vi "FOCUS_V42.vi"(9 "X-pixels":sgl=256.0, 11 "Run":bool) -> (0 "Retrace pixels":sgl, 10 "Pixel Clock (Hz)":sgl)   [LabVIEW 2010] (continued)
      n94 = local write "ScanLineFScope"(sgl[][] [[0.026666667, 0.10555588, 0.18413667, 0.2620946, 0.33912018, 0.4149288, 0.48917702, 0.5616217, 0.6319491, 0.69988036, 0.7651882, 0.8275282, 0.88674605, 0.9425593, 0.9947472, 1.043162, 1.087492, 1.127687, 1.163523, 1.1948596, 1.2216425, 1.2436236, 1.2608614, 1.2732126, 1.2806307, 1.2831601, 1.280641, 1.2732344, 1.2608918, 1.2436653, 1.2216938, 1.1949208, 1.1635948, 1.1277666, 1.0875816, 1.0432596, 0.9948533, 0.9426741, 0.8868671, 0.8276569, 0.7653226, 0.70002097, 0.6320957, 0.5617722, 0.48933217, 0.41508698, 0.33928153, 0.2622585, 0.18430196, 0.10572225, 0.026833316, -0.052056268, -0.13063815, -0.20859744, -0.28562555, -0.36143658, -0.43568876, -0.50813806, -0.57846946, -0.6464066, -0.71171933, -0.77406645, -0.833292, -0.8891114, -0.941308, -0.9897297, -1.0340693, -1.0742743, -1.110118, -1.1414653, -1.1682563, -1.1902486, -1.2074977, -1.2198576, -1.2272873, -1.2298253, -1.2273177, -1.2199228, -1.2075888, -1.1903737, -1.1684103, -1.1416483, -1.110333, -1.0745125, -1.0343375, -0.99002266, -0.9416256, -0.8894551, -0.83365417, -0.7744517, -0.71212274, -0.6468276, -0.57890815, -0.5085887, -0.43615317, -0.36191097, -0.28610873, -0.20908824, -0.13062674, -0.05199747], [-1.2831608, -1.2806358, -1.2732235, -1.2608767, -1.2436445, -1.2216686, -1.1948903, -1.163559, -1.1277268, -1.0875369, -1.0432112, -0.9948003, -0.94261676, -0.88680667, -0.8275926, -0.7652557, -0.69995075, -0.6320225, -0.56169707, -0.48925468, -0.41500804, -0.33920097, -0.26217666, -0.18421942, -0.105639175, -0.026750105, 0.052139297, 0.13072063, 0.20867924, 0.28570607, 0.3615159, 0.4357661, 0.5082131, 0.57854253, 0.6464767, 0.71178705, 0.7741306, 0.83335227, 0.88916856, 0.9413609, 0.9897791, 1.034114, 1.0743139, 1.1101538, 1.1414957, 1.1682826, 1.1902695, 1.2075129, 1.2198684, 1.2272923, 1.2298261, 1.2273127, 1.2199119, 1.2075737, 1.1903529, 1.1683854, 1.1416179, 1.1102973, 1.0744729, 1.034293, 0.98997456, 0.94157284, 0.889398, 0.833594, 0.7743877, 0.7120561, 0.6467577, 0.5788353, 0.50851387, 0.4360761, 0.3618324, 0.28602856, 0.20900682, 0.13105093, 0.052471776, -0.026417017, -0.10530679, -0.18388921, -0.2618492, -0.33887854, -0.4146908, -0.48894495, -0.56139654, -0.63172984, -0.69966996, -0.76498514, -0.82733583, -0.8865652, -0.94238764, -0.9945887, -1.0430137, -1.0873581, -1.127568, -1.1634157, -1.1947683, -1.2215633, -1.2435613, -1.260816, -1.2693994, -1.2762786]] ("transposed array")) -> ()
    }
  }
  n95 = Type Cast(type="" ("name or relative path"), x=w48) -> (*(type *) &x=w45:string)
  n96 = Type Cast(type=tag "" ("6229 Device 2"), x=w65) -> (*(type *) &x=w64:tag)
  n97 = Type Cast(type=refnum<visa-resource-name> " " ("VISA Sutter MP-285"), x=w50) -> (*(type *) &x=w49:refnum<visa-resource-name>)
  n98 = Type Cast(type=refnum<visa-resource-name> refnum ("VISA Sutter MP-285"), x=w54) -> (*(type *) &x=w4:refnum<visa-resource-name>)
  n99 = property on="Run" class="Bool (strict)"("Visible"=w100) -> ()  [unwired: 2 in, 2 out]
  n100 = local write "End experiment"(w101) -> ()
  n101 = property on="colour table" class="Arr (strict)"("Value"=w37) -> ()  [unwired: 2 in, 2 out]
  n102 = property on="Galvos" class="XYGraph (strict)"("X Scale.Range:Minimum"=w3, "X Scale.Range:Maximum"="Scangraph scaling", "Y Scale.Range:Minimum"=w2, "Y Scale.Range:Maximum"="Scangraph scaling") -> ()  [unwired: 2 in, 2 out]
  n103 = Type Cast(type=u16 0 ("Program Version"), x=w84) -> (*(type *) &x=→"Program Version":u16)
  n104 = String To Path(string=w45) -> (path=w44:path)
  n105 = local write "FocusModeSelector"(TRUE ("FocusModeSelector")) -> ()
  n106 = local write "new FreeLine?"(FALSE ("new udl?")) -> ()
  n107 = local write "NewScanpattern"(FALSE ("NewScanpattern")) -> ()
  n108 = local write "VISA XPG-ADC"(w49) -> ()
  n109 = local write "AO/DIO Device"(w67) -> ()
  n110 = local write "VISA Sutter MP-285"(w4) -> ()
  n111 = property on="stop 2" class="Bool (strict)"("Visible"=w100) -> ()  [unwired: 2 in, 2 out]
  n112 = property on="Scan format" class="Ring (strict)"("Disabled"=u8 0) -> ()  [unwired: 2 in, 2 out]
  n113 = local write "AI Device"(w64) -> ()
  n114 = local write "MaiTai setting Path"(w44) -> ()
  n115 = local write "reset?"(125.0 ("reset?")) -> ()
  n116 = property on="Image 2" class="IntGraph (strict)"("Color Table"=w37) -> ()  [unwired: 2 in, 2 out]
  n117 = property on="End experiment" class="Bool (strict)"("Visible"=w100) -> ()  [unwired: 2 in, 2 out]
  n118 = local write "stop 2"(w101) -> ()
  n119 = property on="Hit Graph" class="IntGraph (strict)"("Color Table"=w37) -> ()  [unwired: 2 in, 2 out]
  n120 = while {
    tunnel: w6 -> [w206]
    tunnel: [w161] -> w5
    stop <- w162 stop-if-true
    n121 = flat-sequence {
      tunnel: [w1452] -> w294
      tunnel: w294 -> [w1667]
      tunnel: [w1625] -> w176
      tunnel: [w1640] -> w174
      tunnel: ["Zoom 1 scan voltage"] -> w173
      tunnel: [w1637] -> w172
      tunnel: [w1636] -> w171
      tunnel: [w1621] -> w169
      tunnel: [w1620] -> w168
      tunnel: [w2016] -> w258
      tunnel: [w2015] -> w287
      tunnel: [w1901] -> w289
      tunnel: [w2007] -> w259
      tunnel: [w1962] -> w297
      tunnel: [w1955] -> w261
      tunnel: [w1922] -> w296
      tunnel: [w2013] -> w260
      tunnel: [w2012] -> w284
      tunnel: [w2037] -> w282
      tunnel: [w2030] -> w281
      tunnel: w175 -> [w1886]
      tunnel: w185 -> [w1885]
      tunnel: [w1884] -> w181
      tunnel: w176 -> [w1872]
      tunnel: w174 -> [w1858]
      tunnel: w173 -> [w1871]
      tunnel: w172 -> [w1870]
      tunnel: w171 -> [w1869]
      tunnel: w170 -> [w1867]
      tunnel: w169 -> [w1863]
      tunnel: w168 -> [w1862]
      tunnel: [w1859] -> w167
      frame #0 {
        n122 = property on="Fiberscope" class="TabCtl (strict)"("Visible"="Fiberscope\nMode") -> ()  [unwired: 2 in, 2 out]
        n123 = property on="Hit Graph" class="IntGraph (strict)"("Visible"="Fiberscope\nMode") -> ()  [unwired: 2 in, 2 out]
        n124 = property on="Scale" class="Slide (strict)"("Visible"="Fiberscope\nMode") -> ()  [unwired: 2 in, 2 out]
        n125 = case shown="False" "Fiberscope\nMode" {
          tunnel: ["Mode selector" "Mode selectorFScope"] -> w1452
          frame False {
            n126 = case shown="0, Default" "Scan format" {
              tunnel: [w1558 sgl 64.0 ("X-pixels") sgl 128.0 ("X-pixels") sgl 256.0 ("X-pixels") sgl 512.0 ("X-pixels") sgl 32.0 ("X-pixels")] -> w1483
              tunnel: [w1557 sgl 64.0 ("Y-lines") sgl 128.0 ("Y-lines") sgl 256.0 ("Y-lines") sgl 512.0 ("Y-lines") sgl 32.0 ("Y-lines")] -> w1482
              tunnel: [w1556 sgl 2.0 ("line scan time (ms)") sgl 2.0 ("line scan time (ms)") sgl 2.0 ("line scan time (ms)") sgl 2.0 ("line scan time (ms)") sgl 1.0 ("line scan time (ms)")] -> w1481
              tunnel: [0 2 2 2 2 2] -> w1480
              frame 0, Default {
                n127 = local read "line scan time (ms)"() -> (w1556:sgl)
                n128 = local read "X-pixels"() -> (w1558:sgl)
                n129 = local read "Y-lines"() -> (w1557:sgl)
              }
              frame 1 {
              }
              frame 2 {
              }
              frame 3 {
              }
              frame 4 {
              }
              frame 5 {
              }
            }
            n130 = case shown="0, Default" "Mode selector" {
              tunnel: [2 0 2 2 0 2] -> w1464
              tunnel: [0 1 2 3 1 4] -> w1474
              tunnel: [w1495 w1505 0 w1526 w1536 w1546] -> w1470
              tunnel: w1480 -> [w1495 w1505 _ _ w1536 _]
              tunnel: [0 0 2 2 0 2] -> w1465
              tunnel: [w1500 w1510 u16 0 ("Scan format") u16 0 ("Scan format") w1541 u16 0 ("Scan format")] -> w1479
              tunnel: [TRUE ("Visible") FALSE ("Visible") FALSE ("Visible") FALSE ("Visible") FALSE ("Visible") FALSE ("Visible")] -> w1472
              tunnel: [u8 2 ("Disabled") u8 2 ("Disabled") u8 2 ("Disabled") u8 0 ("Disabled") u8 2 ("Disabled") u8 0 ("Disabled")] -> w1469
              tunnel: [2 2 2 2 2 0] -> w1460
              tunnel: [2 0 0 2 0 2] -> w1463
              tunnel: [w1495 w1505 2 w1526 w1536 w1546] -> w1462
              tunnel: [u8 2 ("Disabled") u8 2 ("Disabled") u8 0 ("Disabled") u8 0 ("Disabled") u8 2 ("Disabled") u8 2 ("Disabled")] -> w1461
              frame 0, Default {
                # "Focus mode"
                n131 = local read "Scan format"() -> (w1500:u16)
              }
              frame 1 {
                # "frame scan"
                n132 = local read "Scan format"() -> (w1510:u16)
              }
              frame 2 {
                # "straight line scan"
              }
              frame 3 {
                w1526 = 2
                # "user-defined line"
              }
              frame 4 {
                # "frame scan piezo"
                n133 = local read "Scan format"() -> (w1541:u16)
              }
              frame 5 {
                w1546 = 2
                # "user-defined line 3D"
              }
            }
            "frame/line indicator" <- w1474
            n134 = Less?(x=w1474, y=u16 3) -> (x < y?=w1476:bool)
            n135 = case shown="False" w1476 {
              tunnel: [TRUE ("Visible") FALSE ("Visible")] -> w1475
              tunnel: [w1487 FALSE ("Visible")] -> w1471
              frame False {
                n136 = property on="Image 3" class="IntGraph (strict)"() -> ("Visible"=w1487:bool)  [unwired: 2 in, 2 out]
              }
              frame True {
              }
            }
            n137 = case shown="3" "Scan format 2" {
              tunnel: [i16 10 ("X-pixels") i16 20 ("X-pixels") i16 40 ("X-pixels") i16 60 ("X-pixels")] -> w1467
              frame 0, Default {
              }
              frame 1 {
              }
              frame 2 {
              }
              frame 3 {
              }
            }
            n138 = local write "X-pixels"(w1483) -> ()
            n139 = local write "Y-lines"(w1482) -> ()
            n140 = local write "line scan time (ms)"(w1481) -> ()
            n141 = property on="phase shift [°]" class="DigNum (strict)"("Disabled"=w1460) -> ()  [unwired: 2 in, 2 out]
            n142 = local write "Scan format"(w1479) -> ()
            n143 = property on="Number of frames" class="DigNum (strict)"("Disabled"=w1463) -> ()  [unwired: 2 in, 2 out]
            n144 = property on="Averaging" class="DigNum (strict)"("Disabled"=w1464) -> ()  [unwired: 2 in, 2 out]
            n145 = property on="z-step (um)" class="DigNum (strict)"("Disabled"=w1464) -> ()  [unwired: 2 in, 2 out]
            n146 = property on="Scan format" class="Ring (strict)"("Disabled"=w1465) -> ()  [unwired: 2 in, 2 out]
            n147 = property on="X-pixels" class="DigNum (strict)"("Disabled"=w1470) -> ()  [unwired: 2 in, 2 out]
            n148 = property on="#" class="DigNum (strict)"("Disabled"=w1470) -> ()  [unwired: 2 in, 2 out]
            n149 = property on="line scan time (ms)" class="DigNum (strict)"("Disabled"=w1470) -> ()  [unwired: 2 in, 2 out]
            n150 = property on="#" class="DigNum (strict)"("Disabled"=w1469) -> ()  [unwired: 2 in, 2 out]
            n151 = property on="Y-lines FreeLine" class="DigNum (strict)"("Disabled"=w1469) -> ()  [unwired: 2 in, 2 out]
            n152 = property on="Y-Scale" class="Bool (strict)"("Disabled"=w1461) -> ()  [unwired: 2 in, 2 out]
            n153 = local write "ImageSelector"(w1471) -> ()
            n154 = property on="XY Graph 1" class="XYGraph (strict)"("Visible"=w1475) -> ()  [unwired: 2 in, 2 out]
            n155 = property on="XY Graph 2" class="XYGraph (strict)"("Visible"=w1475) -> ()  [unwired: 2 in, 2 out]
            n156 = property on="Image 3" class="IntGraph (strict)"("Visible"=w1471) -> ()  [unwired: 2 in, 2 out]
            n157 = property on="Histogram1" class="XYGraph (strict)"("Visible"=w1471) -> ()  [unwired: 2 in, 2 out]
            n158 = property on="Y-lines" class="DigNum (strict)"("Disabled"=w1462) -> ()  [unwired: 2 in, 2 out]
            n159 = Divide(x=4000.0, y=w1467) -> (x/y=→"pixelstoµm":dbl)
            n160 = property on="FocusModeSelector" class="Bool (strict)"("Visible"=w1472) -> ()  [unwired: 2 in, 2 out]
            n161 = property on="XY Graph 3" class="XYGraph (strict)"("Visible"=FALSE) -> ()  [unwired: 2 in, 2 out]
            n162 = property on="XY Graph 4" class="XYGraph (strict)"("Visible"=w1475) -> ()  [unwired: 2 in, 2 out]
            n163 = property on="Image 4" class="IntGraph (strict)"("Visible"=w1471) -> ()  [unwired: 2 in, 2 out]
            n164 = property on="Amplitude Factor" class="DigNum (strict)"("Disabled"=w1460) -> ()  [unwired: 2 in, 2 out]
            n165 = property on="z frequency" class="Slide (strict)"("Disabled"=w1460) -> ()  [unwired: 2 in, 2 out]
            n166 = property on="Histogram2" class="XYGraph (strict)"("Visible"=w1471) -> ()  [unwired: 2 in, 2 out]
            n167 = local write "Open?"(FALSE ("Open?")) -> ()
            n168 = property on="new FreeLine?" class="Bool (strict)"("Disabled"=w1469) -> ()  [unwired: 2 in, 2 out]
            n169 = property on="#" class="DigNum (strict)"("Disabled"=w1463) -> ()  [unwired: 2 in, 2 out]
            n170 = property on="#" class="DigNum (strict)"("Disabled"=w1464) -> ()  [unwired: 2 in, 2 out]
            n171 = property on="Time interval [s]" class="DigNum (strict)"("Disabled"=w1464) -> ()  [unwired: 2 in, 2 out]
            n172 = property on="Number of stacks" class="DigNum (strict)"("Disabled"=w1464) -> ()  [unwired: 2 in, 2 out]
            n173 = property on="#" class="DigNum (strict)"("Disabled"=w1464) -> ()  [unwired: 2 in, 2 out]
            n174 = property on="Cusp Delay" class="DigNum (strict)"("Disabled"=w1465) -> ()  [unwired: 2 in, 2 out]
          }
          frame True {
            n175 = local write "Mode selector"("Mode selectorFScope") -> ()
            n176 = case shown="0, Default" "Mode selectorFScope" {
              tunnel: [u16 2 ("Mode selectorFScope") u16 0 ("Mode selectorFScope") u16 2 ("Mode selectorFScope")] -> w1579
              tunnel: [u16 0 ("Mode selectorFScope") u16 0 ("Mode selectorFScope") u16 2 ("Mode selectorFScope")] -> w1582
              tunnel: [w1593 w1596 u16 0 ("Scan format FScope")] -> w1581
              frame 0, Default {
                n177 = local read "Scan format FScope"() -> (w1593:u16)
              }
              frame 1 {
                n178 = local read "Scan format FScope"() -> (w1596:u16)
              }
              frame 2 {
              }
            }
            n179 = local write "frame/line indicator"("Mode selectorFScope") -> ()
            n180 = local write "Time interval [s]"("Time interval [s]") -> ()
            n181 = local write "Number of stacks"("Number of Stacks") -> ()
            n182 = local read "Number of Frames"() -> (w1588:sgl)
            n183 = case shown="0, Default" "Scan format FScope" {
              tunnel: [w1604 sgl 64.0 ("X dim") sgl 128.0 ("X dim") sgl 256.0 ("X dim") sgl 512.0 ("X dim") sgl 32.0 ("X dim")] -> w1590
              tunnel: [w1603 sgl 64.0 ("Y dim") sgl 128.0 ("Y dim") sgl 256.0 ("Y dim") sgl 512.0 ("Y dim") sgl 32.0 ("Y dim")] -> w1589
              tunnel: [u8 0 ("Disabled") u8 2 ("Disabled") u8 2 ("Disabled") u8 2 ("Disabled") u8 2 ("Disabled") u8 2 ("Disabled")] -> w1591
              frame 0, Default {
                n184 = local read "Y dim"() -> (w1603:sgl)
                n185 = local read "X dim"() -> (w1604:sgl)
              }
              frame 1 {
              }
              frame 2 {
              }
              frame 3 {
              }
              frame 4 {
              }
              frame 5 {
              }
            }
            n186 = local read "Averaging"() -> (w1587:sgl)
            n187 = local write "Scan format FScope"(w1581) -> ()
            n188 = property on="Scan format FScope" class="Ring (strict)"("Disabled"=w1582) -> ()  [unwired: 2 in, 2 out]
            n189 = property on="Time interval [s]" class="DigNum (strict)"("Disabled"=w1579) -> ()  [unwired: 2 in, 2 out]
            n190 = property on="Number of Stacks" class="DigNum (strict)"("Disabled"=w1579) -> ()  [unwired: 2 in, 2 out]
            n191 = property on="Number of Frames" class="DigNum (strict)"("Disabled"=w1579) -> ()  [unwired: 2 in, 2 out]
            n192 = property on="Averaging" class="DigNum (strict)"("Disabled"=w1579) -> ()  [unwired: 2 in, 2 out]
            n193 = property on="#" class="DigNum (strict)"("Disabled"=w1579) -> ()  [unwired: 2 in, 2 out]
            n194 = property on="#" class="DigNum (strict)"("Disabled"=w1579) -> ()  [unwired: 2 in, 2 out]
            n195 = property on="#" class="DigNum (strict)"("Disabled"=w1579) -> ()  [unwired: 2 in, 2 out]
            n196 = local write "X dim"(w1590) -> ()
            n197 = local write "Y dim"(w1589) -> ()
            n198 = property on="Y dim" class="DigNum (strict)"("Disabled"=w1591) -> ()  [unwired: 2 in, 2 out]
            n199 = local write "Number of frames"(w1588) -> ()
            n200 = local write "Averaging"(w1587) -> ()
            n201 = global write "GlobelFSCOPE.vi" "X dim"(w1590) -> ()
            n202 = global write "GlobelFSCOPE.vi" "Y dim"(w1589) -> ()
            n203 = property on="X dim" class="DigNum (strict)"("Disabled"=w1591) -> ()  [unwired: 2 in, 2 out]
            n204 = local write "X-pixels"("X dim") -> ()
            n205 = local write "Y-lines"("Y dim") -> ()
            n206 = global write "GlobelFSCOPE.vi" "Y dim"("Y dim") -> ()
            n207 = global write "GlobelFSCOPE.vi" "X dim"("X dim") -> ()
          }
        }
        n208 = local read "GetFirst"() -> (w1446:bool)
        n209 = local read "GetLast"() -> (w1445:bool)
        n210 = And(x=w1446, y=w1445) -> (x .and. y?=w1444:bool)
        n211 = case shown="True" w1444 {
          frame False {
          }
          frame True {
            n212 = local read "Number of frames"() -> (w1456:sgl)
            n213 = local read "FirstPosition"() -> (w1453:sgl)
            n214 = local read "LastPosition"() -> (w1454:sgl)
            n215 = Decrement(x=w1456) -> (x-1=w1457:sgl)
            n216 = Subtract(x=w1454, y=w1453) -> (x-y=w1458:sgl)
            n217 = Divide(x=w1458, y=w1457) -> (x/y=w1455:sgl)
            n218 = local write "z-step (um)"(w1455) -> ()
          }
        }
        n219 = Get Date/Time String(date format (0)=enum16{"short", "long", "abbreviated"}."abbreviated") -> (time string=→"Time":string)  [unwired: 2 in, 1 out]
        n220 = Format Date/Time String(time format string (%c)="%m%d%y") -> (date/time string=→"Date":string)  [unwired: 2 in]
      }
      frame #1 {
        # "Line scan position and measurement cursors"
        n221 = local read "frame/line indicator"() -> (w1640:u16)
        n222 = Less?(x=w1667, y=3.0) -> (x < y?=w1662:bool)
        n223 = And(x="View line\ncheck box", y=w1662) -> (x .and. y?=w1666:bool)
        n224 = And(x=w1662, y="Measurement cursor check box") -> (x .and. y?=w1661:bool)
        n225 = control-ref of="Image 2"() -> (w1664:refnum<vi>)
        n226 = control-ref of="Image 1"() -> (w1665:refnum<vi>)
        n227 = Divide(x="Y-lines", y="X-pixels") -> (x/y=w1670:sgl)
        n228 = case "Measurement cursor on/off" shown="True" w1661 {
          tunnel: w1664 -> [w1744 w1750]
          tunnel: w1665 -> [w1745 w1751]
          frame False {
            w1743 = FALSE ("Cursor.Visible")
            w1746 = u32 1 ("Active Cursor")
            n229 = property on="OGB value" class="DigNum (strict)"("Visible"=w1743) -> ()  [unwired: 2 in, 2 out]
            n230 = property on="Alexa value" class="DigNum (strict)"("Visible"=w1743) -> ()  [unwired: 2 in, 2 out]
            n231 = property on="Property Node" class="IntGraph (strict)"(reference=w1745, "Active Cursor"=w1746, "Cursor.Visible"=w1743) -> ()  [unwired: 1 in, 2 out]
            n232 = property on="Property Node" class="IntGraph (strict)"(reference=w1744, "Active Cursor"=w1746, "Cursor.Visible"=w1743) -> ()  [unwired: 1 in, 2 out]
          }
          frame True {
            w1747 = u32 1 ("Active Cursor")
            w1752 = u32 16776960
            w1748 = TRUE ("Cursor.Visible")
            w1753 = u32 1 ("Active Cursor")
            n233 = while {
              tunnel: w1751 -> [w1764]
              tunnel: w1750 -> [w1763]
              stop <- w1754 continue-if-true
              w1762 = u32 1 ("Active Cursor")
              n234 = property on="Property Node" class="IntGraph (strict)"(reference=w1764, "Active Cursor"=w1762) -> ("Cursor.Cursor Position:Cursor X"=w1758:dbl, "Cursor.Cursor Position:Cursor Y"=w1756:dbl, "Value"=w1761:u8[][])  [unwired: 1 in, 2 out]
              n235 = Index Array(array=w1761, index (row)=w1758, index (col)=w1756) -> (element=→"OGB value":u8)
              n236 = property on="Property Node" class="IntGraph (strict)"(reference=w1763, "Active Cursor"=w1762, "Cursor.Cursor Position:Cursor X"=w1758, "Cursor.Cursor Position:Cursor Y"=w1756) -> ("Value"=w1757:u8[][])  [unwired: 1 in, 2 out]
              n237 = Index Array(array=w1757, index (row)=w1758, index (col)=w1756) -> (element=→"Alexa value":u8)
              n238 = local read "Measurement cursor check box"() -> (w1755:bool)
              n239 = case shown="False" w1755 {
                selector: w1755 -> [w1765 w1767]
                tunnel: [w1765 w1767] -> w1754
                frame False {
                  n240 = property on="Run" class="Bool (strict)"("Disabled"=u8 0) -> ()  [unwired: 2 in, 2 out]
                }
                frame True {
                }
              }
            }
            n241 = property on="Run" class="Bool (strict)"("Disabled"=u8 2) -> ()  [unwired: 2 in, 2 out]
            n242 = property on="Property Node" class="IntGraph (strict)"(reference=w1751, "Active Cursor"=w1753, "Cursor.Visible"=w1748, "Cursor.Cursor Color"=w1752, "Cursor.Cursor Position:Cursor X"=w1747, "Cursor.Cursor Position:Cursor Y"=w1747) -> ()  [unwired: 1 in, 2 out]
            n243 = property on="Property Node" class="IntGraph (strict)"(reference=w1750, "Active Cursor"=w1753, "Cursor.Visible"=w1748, "Cursor.Cursor Color"=w1752) -> ()  [unwired: 1 in, 2 out]
            n244 = property on="OGB value" class="DigNum (strict)"("Visible"=w1748) -> ()  [unwired: 2 in, 2 out]
            n245 = property on="Alexa value" class="DigNum (strict)"("Visible"=w1748) -> ()  [unwired: 2 in, 2 out]
          }
        }
        n246 = Greater?(x=w1670, y=1.0) -> (0:w1671:bool)
        n247 = local read "Fiberscope\nMode"() -> (w1645:bool)
        n248 = case shown="True" w1645 {
          tunnel: [w1684 w1685] -> w1659
          frame False {
            n249 = local read "Mode selector"() -> (w1684:u16)
          }
          frame True {
            n250 = local read "Mode selectorFScope"() -> (w1685:u16)
          }
        }
        n251 = case shown="False" w1671 {
          tunnel: w1670 -> [w1774 _]
          tunnel: [w1773 w1813] -> w1653
          tunnel: [w1771 w1812] -> w1652
          tunnel: [w1770 w1811] -> w1651
          frame False {
            w1769 = u32 512 ("Plot Area:Size:Width")
            n252 = Multiply(x=w1769, y=w1774) -> (x*y=w1768:sgl)
            n253 = property on="Image 1" class="IntGraph (strict)"("Plot Area:Size:Width"=w1769, "Plot Area:Size:Height"=w1768) -> ()  [unwired: 2 in, 2 out]
            n254 = property on="Image 2" class="IntGraph (strict)"("Plot Area:Size:Width"=w1769, "Plot Area:Size:Height"=w1768) -> ()  [unwired: 2 in, 2 out]
            n255 = property on="ImageSlide" class="Slide (strict)"("Housing Size:Height"=w1768) -> ()  [unwired: 2 in, 2 out]
            n256 = property on="XY Graph 1" class="XYGraph (strict)"("Plot Area:Size:Width"=w1769, "Plot Area:Size:Height"=w1768) -> ()  [unwired: 2 in, 2 out]
            n257 = property on="XY Graph 2" class="XYGraph (strict)"("Plot Area:Size:Width"=w1769, "Plot Area:Size:Height"=w1768) -> ()  [unwired: 2 in, 2 out]
            n258 = property on="SlideHorizontal" class="Slide (strict)"("Housing Size:Width"=w1769) -> ()  [unwired: 2 in, 2 out]
            n259 = property on="XY Graph 3" class="XYGraph (strict)"("Plot Area:Size:Width"=w1769, "Plot Area:Size:Height"=w1768) -> ()  [unwired: 2 in, 2 out]
            n260 = property on="XY Graph 4" class="XYGraph (strict)"("Plot Area:Size:Width"=w1769, "Plot Area:Size:Height"=w1768) -> ()  [unwired: 2 in, 2 out]
            n261 = local read "frame/line indicator"() -> (w1772:u16)
            n262 = case shown="2" w1772 {
              tunnel: [FALSE ("Visible") w1781 w1791 w1795 w1804] -> w1773
              tunnel: [_ w1779 w1788 w1796 w1802] -> w1771
              tunnel: [FALSE ("Visible") FALSE ("Visible") FALSE ("Visible") FALSE ("Visible") TRUE ("Visible")] -> w1770
              frame 0, Default {
              }
              frame 1 {
                n263 = local read "Number of frames"() -> (w1778:sgl)
                n264 = Decrement(x=w1778) -> (x-1=w1779:sgl)
                n265 = Less Or Equal To 0?(x=w1779) -> (x <= 0?=w1780:bool)
                n266 = case shown="False" w1780 {
                  tunnel: [TRUE ("Visible") FALSE ("Visible")] -> w1781
                  frame False {
                  }
                  frame True {
                  }
                }
              }
              frame 2 {
                n267 = local read "Y-lines"() -> (w1786:sgl)
                n268 = local read "Number of frames"() -> (w1784:sgl)
                n269 = Multiply(x=w1786, y=w1784) -> (x*y=w1785:sgl)
                n270 = local read "X-pixels"() -> (w1790:sgl)
                n271 = Subtract(x=w1785, y=w1790) -> (x-y=w1788:sgl)
                n272 = Less Or Equal To 0?(x=w1788) -> (x <= 0?=w1789:bool)
                n273 = case shown="False" w1789 {
                  tunnel: [TRUE ("Visible") FALSE ("Visible")] -> w1791
                  frame False {
                  }
                  frame True {
                  }
                }
              }
              frame 3 {
                n274 = local read "X-pixels FreeLine"() -> (w1798:sgl)
                n275 = local read "Y-lines FreeLine"() -> (w1799:sgl)
                n276 = Subtract(x=w1799, y=w1798) -> (x-y=w1796:sgl)
                n277 = Less Or Equal To 0?(x=w1796) -> (x <= 0?=w1797:bool)
                n278 = case shown="True" w1797 {
                  tunnel: [TRUE ("Visible") FALSE ("Visible")] -> w1795
                  frame False {
                  }
                  frame True {
                  }
                }
              }
              frame 4 {
                n279 = local read "X-pixels FreeLine"() -> (w1806:sgl)
                n280 = local read "Y-lines FreeLine"() -> (w1807:sgl)
                n281 = Subtract(x=w1807, y=w1806) -> (x-y=w1802:sgl)
                n282 = Less Or Equal To 0?(x=w1802) -> (x <= 0?=w1805:bool)
                n283 = case shown="True" w1805 {
                  tunnel: [FALSE ("Visible") FALSE ("Visible")] -> w1804
                  frame False {
                  }
                  frame True {
                  }
                }
              }
            }
          }
          frame True {
            w1810 = 512
            n284 = property on="Image 1" class="IntGraph (strict)"("Plot Area:Size:Width"=w1810, "Plot Area:Size:Height"=w1810) -> ()  [unwired: 2 in, 2 out]
            n285 = property on="Image 2" class="IntGraph (strict)"("Plot Area:Size:Width"=w1810, "Plot Area:Size:Height"=w1810) -> ()  [unwired: 2 in, 2 out]
            n286 = property on="ImageSlide" class="Slide (strict)"("Housing Size:Height"=w1810) -> ()  [unwired: 2 in, 2 out]
            n287 = property on="XY Graph 1" class="XYGraph (strict)"("Plot Area:Size:Width"=w1810, "Plot Area:Size:Height"=w1810) -> ()  [unwired: 2 in, 2 out]
            n288 = property on="XY Graph 2" class="XYGraph (strict)"("Plot Area:Size:Width"=w1810, "Plot Area:Size:Height"=w1810) -> ()  [unwired: 2 in, 2 out]
            n289 = property on="SlideHorizontal" class="Slide (strict)"("Housing Size:Width"=w1810) -> ()  [unwired: 2 in, 2 out]
            n290 = local read "frame/line indicator"() -> (w1814:u16)
            n291 = property on="XY Graph 4" class="XYGraph (strict)"("Plot Area:Size:Width"=w1810, "Plot Area:Size:Height"=w1810) -> ()  [unwired: 2 in, 2 out]
            n292 = property on="XY Graph 3" class="XYGraph (strict)"("Plot Area:Size:Width"=w1810, "Plot Area:Size:Height"=w1810) -> ()  [unwired: 2 in, 2 out]
            n293 = case shown="2" w1814 {
              tunnel: [FALSE ("Visible") w1820 w1830 w1837 w1845] -> w1813
              tunnel: [_ w1821 w1831 w1836 w1844] -> w1812
              tunnel: [FALSE ("Visible") FALSE ("Visible") FALSE ("Visible") FALSE ("Visible") TRUE ("Visible")] -> w1811
              frame 0, Default {
                n294 = One Button Dialog(message="Unable to display the whole image using these settings.\nThe requested image can be acquired and saved, but\n      the displayed image will be clipped.\nThis is because the y-dimension (# lines) is larger\n      than the x-dimension (# pixels).\nTo solve this problem, switch the values of x- and y-\n      dimensions (and rotate the image, if necessary).") -> ()  [unwired: 1 in, 1 out]
              }
              frame 1 {
                n295 = local read "Number of frames"() -> (w1819:sgl)
                n296 = Decrement(x=w1819) -> (x-1=w1821:sgl)
                n297 = Less Or Equal To 0?(x=w1821) -> (x <= 0?=w1822:bool)
                n298 = case shown="False" w1822 {
                  tunnel: [TRUE ("Visible") FALSE ("Visible")] -> w1820
                  frame False {
                  }
                  frame True {
                  }
                }
              }
              frame 2 {
                n299 = local read "Y-lines"() -> (w1827:sgl)
                n300 = local read "Number of frames"() -> (w1826:sgl)
                n301 = local read "X-pixels"() -> (w1829:sgl)
                n302 = Multiply(x=w1827, y=w1826) -> (x*y=w1825:sgl)
                n303 = Subtract(x=w1825, y=w1829) -> (x-y=w1831:sgl)
                n304 = Less Or Equal To 0?(x=w1831) -> (x <= 0?=w1832:bool)
                n305 = case shown="False" w1832 {
                  tunnel: [TRUE ("Visible") FALSE ("Visible")] -> w1830
                  frame False {
                  }
                  frame True {
                  }
                }
              }
              frame 3 {
                n306 = local read "X-pixels FreeLine"() -> (w1839:sgl)
                n307 = local read "Y-lines FreeLine"() -> (w1840:sgl)
                n308 = Subtract(x=w1840, y=w1839) -> (x-y=w1836:sgl)
                n309 = Less Or Equal To 0?(x=w1836) -> (x <= 0?=w1838:bool)
                n310 = case shown="False" w1838 {
                  tunnel: [TRUE ("Visible") FALSE ("Visible")] -> w1837
                  frame False {
                  }
                  frame True {
                  }
                }
              }
              frame 4 {
                n311 = local read "X-pixels FreeLine"() -> (w1847:sgl)
                n312 = local read "Y-lines FreeLine"() -> (w1848:sgl)
                n313 = Subtract(x=w1848, y=w1847) -> (x-y=w1844:sgl)
                n314 = Less Or Equal To 0?(x=w1844) -> (x <= 0?=w1846:bool)
                n315 = case shown="False" w1846 {
                  tunnel: [FALSE ("Visible") FALSE ("Visible")] -> w1845
                  frame False {
                  }
                  frame True {
                  }
                }
              }
            }
          }
        }
        "ImageSlideMax" <- w1652
        n316 = Bundle("frame/line indicator"=w1640, "X-pixels"="X-pixels", "Y-lines"="Y-lines", "line scan time (ms)"="line scan time (ms)", "Zoom 1 scan voltage"="Zoom 1 scan voltage", "Scanblock Factor"="Scanblock Factor", "Scanpattern"="Scanpattern") -> (w1635:T13)  [unwired: 1 in]
        n317 = case "Cursors to indicate line scan position" shown="True" w1666 {
          tunnel: w1665 -> [w1731 w1735]
          tunnel: w1664 -> [w1730 w1734]
          frame False {
            w1732 = FALSE ("Cursor.Visible")
            w1733 = u32 0 ("Active Cursor")
            n318 = property on="Property Node" class="IntGraph (strict)"(reference=w1731, "Active Cursor"=w1733, "Cursor.Visible"=w1732) -> ()  [unwired: 1 in, 2 out]
            n319 = property on="Property Node" class="IntGraph (strict)"(reference=w1730, "Active Cursor"=w1733, "Cursor.Visible"=w1732) -> ()  [unwired: 1 in, 2 out]
          }
          frame True {
            w1739 = u32 14418136
            w1742 = TRUE ("Cursor.Visible")
            w1741 = -1.0 ("Cursor.Cursor Position:Cursor X")
            w1740 = u32 0 ("Active Cursor")
            n320 = local read "Y-lines"() -> (w1736:sgl)
            n321 = Divide(x=w1736, y=2.0) -> (x/y=w1737:dbl)
            n322 = property on="Property Node" class="IntGraph (strict)"(reference=w1735, "Active Cursor"=w1740, "Cursor.Cursor Position:Cursor X"=w1741, "Cursor.Cursor Position:Cursor Y"=w1737, "Cursor.Visible"=w1742, "Cursor.Cursor Color"=w1739) -> ()  [unwired: 1 in, 2 out]
            n323 = property on="Property Node" class="IntGraph (strict)"(reference=w1734, "Active Cursor"=w1740, "Cursor.Cursor Position:Cursor X"=w1741, "Cursor.Cursor Position:Cursor Y"=w1737, "Cursor.Visible"=w1742, "Cursor.Cursor Color"=w1739) -> ()  [unwired: 1 in, 2 out]
          }
        }
        n324 = case shown="2" w1659 {
          tunnel: "X-pixels" -> [w1686 w1709 w1712 w1729]
          tunnel: "Y-lines" -> [w1687 w1708 _ w1728]
          tunnel: "X-pixels" -> [w1697 w1707 w1713 w1727]
          tunnel: "Y-lines" -> [w1696 w1706 _ w1726]
          tunnel: [0.0 ("X Scale.Range:Minimum") 0.0 ("X Scale.Range:Minimum") 0.0 ("X Scale.Range:Minimum") 0.0 ("X Scale.Range:Minimum")] -> w1649
          tunnel: [w1694 w1704 w1711 w1724] -> w1648
          tunnel: [0.0 ("Y Scale.Range:Minimum") 0.0 ("Y Scale.Range:Minimum") 0.0 ("Y Scale.Range:Minimum") 0.0 ("Y Scale.Range:Minimum")] -> w1647
          tunnel: [w1692 w1702 w1711 w1722] -> w1646
          tunnel: [0.0 ("X Scale.Range:Minimum") 0.0 ("X Scale.Range:Minimum") 0.0 ("X Scale.Range:Minimum") 0.0 ("X Scale.Range:Minimum")] -> w1658
          tunnel: [w1690 w1700 w1710 w1720] -> w1657
          tunnel: [0.0 ("Y Scale.Range:Minimum") 0.0 ("Y Scale.Range:Minimum") 0.0 ("Y Scale.Range:Minimum") 0.0 ("Y Scale.Range:Minimum")] -> w1656
          tunnel: [w1688 w1698 w1710 w1718] -> w1654
          frame 0, Default {
            n325 = Decrement(x=w1686) -> (x-1=w1694:sgl)
            n326 = Decrement(x=w1687) -> (x-1=w1692:sgl)
            n327 = Decrement(x=w1697) -> (x-1=w1690:sgl)
            n328 = Decrement(x=w1696) -> (x-1=w1688:sgl)
          }
          frame 1 {
            n329 = Decrement(x=w1709) -> (x-1=w1704:sgl)
            n330 = Decrement(x=w1708) -> (x-1=w1702:sgl)
            n331 = Decrement(x=w1707) -> (x-1=w1700:sgl)
            n332 = Decrement(x=w1706) -> (x-1=w1698:sgl)
          }
          frame 2 {
            n333 = Decrement(x=w1712) -> (x-1=w1711:sgl)
            n334 = Decrement(x=w1713) -> (x-1=w1710:sgl)
          }
          frame 4 {
            n335 = Decrement(x=w1729) -> (x-1=w1724:sgl)
            n336 = Decrement(x=w1728) -> (x-1=w1722:sgl)
            n337 = Decrement(x=w1727) -> (x-1=w1720:sgl)
            n338 = Decrement(x=w1726) -> (x-1=w1718:sgl)
          }
        }
        n339 = case shown="True" "Scanpattern" {
          tunnel: [w1678 w1683] -> w1642
          tunnel: [w1677 w1682] -> w1637
          tunnel: [w1676 w1681] -> w1636
          tunnel: w1635 -> [w1675 w1680]
          tunnel: [w1674 w1679] -> w1621
          frame True {
            n340 = call "ScanGeniFOCUS.vi"("Parameters In"=w1675) -> ("X-Scansignals"=w1677:dbl[], "Parameters out"=w1678:T14, "Y-Scansignals"=w1676:dbl[], "Z-Scansignals"=w1674:dbl[])
          }
          frame False {
            n341 = call "ScanGeniFOCUS.vi"("Parameters In"=w1680) -> ("X-Scansignals"=w1682:dbl[], "Parameters out"=w1683:T14, "Y-Scansignals"=w1681:dbl[], "Z-Scansignals"=w1679:dbl[])
          }
        }
        n342 = Unbundle(w1642) -> ("Scan mode"=w1622:u16, "Pixel Clock (Hz)"=→"Pixel Clock (Hz)":sgl, "pixel dwell time [us]"=w1625:sgl, "Frame rate (Hz)"=→"Frame rate [Hz]":sgl, "total x pixels"=→"total x pixels":sgl, "total y lines"=→"total y pixels":sgl, "Retrace pixels (tdown)"=→"Retrace pixels":sgl, "Scan Cut-Off (either end)"=→"Scan Cut-Off (either end)":sgl, "pixels in frame"=→"pixels in frame":sgl, "pixels in frame + yretrace"=→"pixels in frame + yretrace":sgl, "Scanblock length"=→"Scan Block Length":sgl, "total pixels in frame"=→"total pixels in frame":sgl, "Z-scan mode"=w1620:u16)
        "pixel dwell time [us]" <- w1625
        "Scan mode" <- w1622
        n343 = property on="Image 1" class="IntGraph (strict)"("X Scale.Range:Minimum"=w1649, "X Scale.Range:Maximum"=w1648, "Y Scale.Range:Minimum"=w1647, "Y Scale.Range:Maximum"=w1646) -> ()  [unwired: 2 in, 2 out]
        n344 = property on="Image 2" class="IntGraph (strict)"("X Scale.Range:Minimum"=w1658, "X Scale.Range:Maximum"=w1657, "Y Scale.Range:Minimum"=w1656, "Y Scale.Range:Maximum"=w1654) -> ()  [unwired: 2 in, 2 out]
        n345 = property on="Hit Graph" class="IntGraph (strict)"("X Scale.Range:Minimum"=w1649, "X Scale.Range:Maximum"=w1648, "Y Scale.Range:Minimum"=w1647, "Y Scale.Range:Maximum"=w1646) -> ()  [unwired: 2 in, 2 out]
        n346 = case shown="0, Default" w1622 {
          frame 1 {
            n347 = property on="Shift" class="DigNum (strict)"("Visible"=TRUE) -> ()  [unwired: 2 in, 2 out]
          }
          frame 0, Default {
            n348 = property on="Shift" class="DigNum (strict)"("Visible"=FALSE) -> ()  [unwired: 2 in, 2 out]
          }
        }
        n349 = Not(x=w1651) -> (.not. x?=w1650:bool)
        n350 = local write "XScale"(w1650) -> ()
        n351 = property on="SlideHorizontal" class="Slide (strict)"("Visible"=w1651) -> ()  [unwired: 2 in, 2 out]
        n352 = property on="ImageSlide" class="Slide (strict)"("Scale.Range:Minimum"=0.0, "Scale.Range:Maximum"=w1652) -> ()  [unwired: 2 in, 2 out]
        n353 = property on="ImageSlide" class="Slide (strict)"("Visible"=w1653) -> ()  [unwired: 2 in, 2 out]
        n354 = property on="Play Movie" class="Bool (strict)"("Visible"=w1653) -> ()  [unwired: 2 in, 2 out]
        n355 = property on="Velocity" class="Slide (strict)"("Visible"=w1653) -> ()  [unwired: 2 in, 2 out]
      }
      frame #2 {
        w1958 = 10123 items=["Finite Samples"=10178, "Continuous Samples"=10123, "Hardware Timed Single Point"=12522] ("sample mode")
        w2011 = 10123 items=["Finite Samples"=10178, "Continuous Samples"=10123, "Hardware Timed Single Point"=12522] ("sample mode")
        w2019 = 10123 items=["Finite Samples"=10178, "Continuous Samples"=10123, "Hardware Timed Single Point"=12522] ("sample mode")
        w2033 = 2.0 ("Y Scale.Range:Maximum")
        w2034 = 1.0 ("Y Scale.Range:Minimum")
        w2035 = 0.0 ("X Scale.Range:Minimum")
        # "x-y plot of galvo signals"
        n356 = local read "frame/line indicator"() -> (w2028:u16)
        n357 = case shown="4" w2028 {
          tunnel: [w2987 w2988 w2990 w2992 w3004] -> w2032
          tunnel: [w2986 w2989 w2991 w2992 w2996] -> w2031
          frame 0, Default {
            n358 = property on="Image 3" class="IntGraph (strict)"() -> ("X Scale.Range:Maximum"=w2987:dbl, "Y Scale.Range:Maximum"=w2986:dbl)  [unwired: 2 in, 2 out]
          }
          frame 1 {
            n359 = property on="Image 3" class="IntGraph (strict)"() -> ("X Scale.Range:Maximum"=w2988:dbl, "Y Scale.Range:Maximum"=w2989:dbl)  [unwired: 2 in, 2 out]
          }
          frame 2 {
            n360 = property on="Image 3" class="IntGraph (strict)"() -> ("X Scale.Range:Maximum"=w2990:dbl, "Y Scale.Range:Maximum"=w2991:dbl)  [unwired: 2 in, 2 out]
          }
          frame 3 {
            n361 = local read "X-pixels FreeLine"() -> (w2993:sgl)
            n362 = Decrement(x=w2993) -> (x-1=w2992:sgl)
          }
          frame 4 {
            w2999 = sgl 1000000.0 ("y")
            n363 = local read "XScale"() -> (w3003:bool)
            n364 = local read "X-pixels FreeLine"() -> (w2994:sgl)
            n365 = case shown="True" w3003 {
              tunnel: [w3009 w3013] -> w3004
              tunnel: [w3009 w3012] -> w2995
              tunnel: [w3008 sgl 0.0] -> w3001
              tunnel: [TRUE ("XScale") FALSE ("XScale")] -> w3005
              tunnel: w2994 -> [w3006 _]
              frame False {
                n366 = local read "Y-lines FreeLine"() -> (w3009:sgl)
                n367 = Subtract(x=w3006, y=w3009) -> (x-y=w3008:sgl)
              }
              frame True {
                n368 = local read "X-pixels FreeLine"() -> (w3013:sgl)
                n369 = local read "Y-lines FreeLine"() -> (w3012:sgl)
              }
            }
            n370 = property on="SlideHorizontal" class="Slide (strict)"("Visible"=w3005) -> ()  [unwired: 2 in, 2 out]
            n371 = property on="SlideHorizontal" class="Slide (strict)"("Scale.Range:Minimum"=0.0, "Scale.Range:Maximum"=w3001) -> ()  [unwired: 2 in, 2 out]
            n372 = Divide(x=w2999, y=w2994) -> (x/y=w3000:sgl)
            n373 = Multiply(x=w2995, y=w2994) -> (x*y=w2998:sgl)
            n374 = Greater?(x=w2998, y=w2999) -> (0:w2997:bool)
            n375 = Select(t=w3000, s=w2997, f=w2995) -> (s? t:f=w2996:sgl)
          }
        }
        n376 = property on="Image 2" class="IntGraph (strict)"() -> ("Color Table"=w2036:u32[])  [unwired: 2 in, 2 out]
        n377 = property on="Histogram1" class="XYGraph (strict)"("Y Scale.Range:Minimum"=w2034, "Y Scale.Range:Maximum"=w2033) -> ()  [unwired: 2 in, 2 out]
        n378 = local read "Fiberscope\nMode"() -> (w1894:bool)
        n379 = Greater Or Equal?(x=w1858, y=u16 3) -> (x >= y?=w1856:bool)
        n380 = property on="Image 3" class="IntGraph (strict)"("X Scale.Range:Minimum"=w2035, "X Scale.Range:Maximum"=w2032, "Y Scale.Range:Minimum"=w2035, "Y Scale.Range:Maximum"=w2031, "Color Table"=w2036) -> ()  [unwired: 2 in, 2 out]
        n381 = property on="Image 4" class="IntGraph (strict)"("X Scale.Range:Minimum"=w2035, "X Scale.Range:Maximum"=w2032, "Y Scale.Range:Minimum"=w2035, "Y Scale.Range:Maximum"=w2031, "Color Table"=w2036) -> ()  [unwired: 2 in, 2 out]
        n382 = property on="Histogram2" class="XYGraph (strict)"("Y Scale.Range:Minimum"=w2034, "Y Scale.Range:Maximum"=w2033) -> ()  [unwired: 2 in, 2 out]
        n383 = local write "Scanpattern"(FALSE ("Scanpattern")) -> ()
        n384 = property on="Histogram1" class="XYGraph (strict)"("X Scale.Range:Minimum"=w2035, "X Scale.Range:Maximum"=w2032) -> ()  [unwired: 2 in, 2 out]
        n385 = property on="Histogram2" class="XYGraph (strict)"("X Scale.Range:Minimum"=w2035, "X Scale.Range:Maximum"=w2032) -> ()  [unwired: 2 in, 2 out]
        n386 = case shown="True" w1856 {
          tunnel: [w2046 w2047] -> w1855
          frame False {
            n387 = local read "pixel dwell time [us]"() -> (w2046:sgl)
          }
          frame True {
            n388 = local read "pixel dwell time [us] FreeLine"() -> (w2047:sgl)
          }
        }
        n389 = local read "Mode selectorFScope"() -> (w1891:u16)
        n390 = local read "#"() -> (w1864:sgl)
        n391 = Array Subset(array=w1867, length (col)=w1864) -> (w1866:u8[][])  [unwired: 3 in]
        n392 = flat-sequence {
          tunnel: [w2985] -> w1921
          frame #0 {
            n393 = call <vilib>:"DAQmx Reset Device.vi"("device in"="AO/DIO Device") -> ("error out"=w2984:errorcluster)  [unwired: 14 in]
            n394 = call <vilib>:"DAQmx Reset Device.vi"("device in"="AI Device", "error in"=w2984) -> ("error out"=w2985:errorcluster)  [unwired: 13 in]
          }
        }
        n395 = local read "AO/DIO Device"() -> (w1941:tag)
        n396 = local read "AO/DIO Device"() -> (w1945:tag)
        n397 = case shown="True" "Test Run?" {
          tunnel: w1866 -> [_ w2048]
          frame False {
          }
          frame True {
            "Image3Arrayd" <- w2048
          }
        }
        n398 = Concatenate Strings(tag "/" ("destination terminal"), w1941, tag "/ao/SampleClock" ("source of ticks")) -> (w1942:string)
        n399 = Concatenate Strings(w1945, tag "/ctr0" ("counter")) -> (w1943:string)
        n400 = Type Cast(type=tag "" ("source of ticks"), x=w1942) -> (*(type *) &x=w1937:tag)
        n401 = Type Cast(type=tag "" ("counter"), x=w1943) -> (*(type *) &x=w1925:tag)
        n402 = local read "frame/line indicator"() -> (w1918:u16)
        n403 = local read "AO/DIO Device"() -> (w2000:tag)
        n404 = case shown="False" w1894 {
          tunnel: w1871 -> [w2105 _]
          tunnel: w1858 -> [w2104 _]
          tunnel: "new FreeLine?" -> [w2103 _]
          tunnel: [w2102 FALSE ("XScale")] -> w1861
          tunnel: [w2101 w2859] -> w2014
          tunnel: [w2100 w2852] -> w2004
          tunnel: [w2099 w2862] -> w1887
          tunnel: w2000 -> [w2098 w2857]
          tunnel: tag "" ("physical channels") -> [w2097 w2858]
          tunnel: [w2096 w2855] -> w1878
          tunnel: [w2095 sgl 1.0 ("total y pixels")] -> w1952
          tunnel: [w2094 w2855] -> w1946
          tunnel: [w2093 w2854] -> w1914
          tunnel: w1891 -> [_ w2853]
          tunnel: w1886 -> [w2092 _]
          tunnel: w1885 -> [w2091 _]
          tunnel: w1872 -> [w2090 _]
          tunnel: w1870 -> [w2089 _]
          tunnel: w1869 -> [w2088 _]
          tunnel: w1863 -> [w2087 _]
          tunnel: w1862 -> [w2086 _]
          tunnel: [w2085 FALSE ("XScale")] -> w1860
          tunnel: [w2084 _] -> w1859
          frame False {
            n405 = case shown="0, Default" w2104 {
              tunnel: w2105 -> [_ _ _ w2595 w2699]
              tunnel: [w2174 w2269 w2468 w2590 w2698] -> w2100
              tunnel: [w2187 w2290 w2460 w2593 w2697] -> w2094
              tunnel: [w2189 w2294 w2462 w2592 w2696] -> w2096
              tunnel: [w2177 w2293 w2463 w2594 w2700] -> w2095
              tunnel: w2103 -> [_ _ _ w2591 w2694]
              tunnel: [w2186 w2269 w2468 w2590 w2698] -> w2099
              tunnel: [FALSE ("XScale") FALSE ("XScale") FALSE ("XScale") FALSE ("XScale") TRUE ("XScale")] -> w2102
              tunnel: [w2172 w2264 w2526 w2583 w2686] -> w2101
              tunnel: w2098 -> [w2110 w2268 w2527 w2585 w2688]
              tunnel: w2097 -> [w2173 w2267 w2528 w2584 w2687]
              tunnel: [w2171 w2292 w2461 w2580 w2684] -> w2093
              tunnel: w2092 -> [_ _ _ _ w2683]
              tunnel: w2091 -> [_ _ _ _ w2682]
              tunnel: w2090 -> [_ w2291 _ _ _]
              tunnel: w2089 -> [w2169 w2354 w2458 w2578 w2681]
              tunnel: w2088 -> [w2168 w2353 w2455 w2579 w2680]
              tunnel: w2087 -> [w2167 w2352 w2521 _ _]
              tunnel: w2086 -> [_ _ _ _ _]
              tunnel: [FALSE ("XScale") FALSE ("XScale") TRUE ("XScale") FALSE ("XScale") FALSE ("XScale")] -> w2085
              tunnel: [w2106 w2275 _ _ _] -> w2084
              frame 0, Default {
                w2170 = 10123 items=["Finite Samples"=10178, "Continuous Samples"=10123, "Hardware Timed Single Point"=12522] ("sample mode")
                n406 = local read "On?"() -> (w2114:bool)
                n407 = local read "[µm] per pixel at zoom 1"() -> (w2119:sgl)
                n408 = local read "Y-lines"() -> (w2118:sgl)
                n409 = local read "Rotation z"() -> (w2113:sgl)
                n410 = case shown="False" w2114 {
                  tunnel: w2113 -> [_ w2236]
                  tunnel: [sgl 0.0 ("Rotation z") w2236] -> w2112
                  frame False {
                  }
                  frame True {
                  }
                }
                n411 = Divide(x=w2112, y=360.0) -> (x/y=w2165:dbl)
                n412 = Multiply(x=w2165, y=6.283185307179586) -> (x*y=w2163:dbl)
                n413 = Build Array(w2169, w2168, w2167) -> (w2149:dbl[][])
                "OriginalScanSignals" <- w2149
                n414 = Sine(x=w2163) -> (sin(x)=w2122:dbl)
                n415 = Cosine(x=w2163) -> (cos(x)=w2162:dbl)
                n416 = Multiply(x=w2119, y=w2118) -> (x*y=w2116:sgl)
                n417 = Negate(x=w2122) -> (-x=w2161:dbl)
                n418 = Array Subset(array=w2149, length (row)=1 ("length")) -> (w2152:dbl[][])  [unwired: 3 in]
                n419 = Array Subset(array=w2149, index (row)=1 ("index")) -> (w2156:dbl[][])  [unwired: 3 in]
                n420 = local read "Zoom"() -> (w2123:sgl)
                n421 = Build Array(w2122, w2162) -> (w2158:dbl[])
                n422 = Build Array(w2162, w2161) -> (w2159:dbl[])
                n423 = local read "total y pixels"() -> (w2177:sgl)
                n424 = Build Array(w2159, w2158) -> (w2157:dbl[][])
                n425 = local read "Rotation"() -> (w2179:sgl)
                n426 = call-poly <vilib>:"A x B.vi"("B"=w2156, "A"=w2157) -> ("A x B"=w2150:T15)  [unwired: 1 out]
                n427 = local read "Position piezo [µm]"() -> (w2121:sgl)
                n428 = Divide(x=w2116, y=w2123) -> (x/y=w2127:sgl)
                n429 = local read "total x pixels"() -> (w2189:sgl)
                n430 = Divide(x=w2127, y=sgl 40.0) -> (x/y=w2133:sgl)
                n431 = Multiply(x=w2179, y=-1.0) -> (x*y=w2182:dbl)
                n432 = Index Array(array=w2150, index (row)=0 ("disabled index (col)")) -> (element=w2151:dbl[])  [unwired: 1 in]
                n433 = Index Array(array=w2150, index (row)=1 ("disabled index (col)")) -> (element=w2124:dbl[])  [unwired: 1 in]
                n434 = Array Max & Min(array=w2124) -> (max value=w2125:dbl, min value=w2130:dbl)  [unwired: 2 out]
                n435 = Subtract(x=w2125, y=w2130) -> (x-y=w2132:dbl)
                n436 = Equal To 0?(x=w2132) -> (x = 0?=w2135:bool)
                n437 = Subtract(x=w2124, y=w2130) -> (x-y=w2136:dbl[])
                n438 = Subtract(x=w2182, y=360.0) -> (x-y=w2180:dbl)
                n439 = local read "FocusModeSelector"() -> (w2109:bool)
                n440 = Multiply(x=w2133, y=w2122) -> (x*y=w2134:dbl)
                n441 = Divide(x=w2180, y=360.0) -> (x/y=w2195:dbl)
                n442 = Build Array (concatenate)(w2152, w2151) -> (w2148:dbl[][])
                n443 = Divide(x=w2121, y=sgl 40.0) -> (x/y=w2117:sgl)
                n444 = case shown="False" w2135 {
                  tunnel: [w2249 w2250] -> w2131
                  tunnel: w2132 -> [w2248 _]
                  tunnel: w2134 -> [w2246 _]
                  tunnel: w2117 -> [w2244 w2252]
                  tunnel: w2136 -> [w2238 w2251]
                  frame False {
                    n445 = Divide(x=w2238, y=w2248) -> (x/y=w2247:dbl[])
                    n446 = Multiply(x=w2247, y=w2246) -> (x*y=w2245:dbl[])
                    n447 = Add(x=w2245, y=w2244) -> (x+y=w2237:dbl[])
                    n448 = Array Max & Min(array=w2237) -> (max value=w2243:dbl, min value=w2240:dbl)  [unwired: 2 out]
                    n449 = Subtract(x=w2243, y=w2240) -> (x-y=w2242:dbl)
                    n450 = Divide(x=w2242, y=2.0) -> (x/y=w2239:dbl)
                    n451 = Subtract(x=w2237, y=w2239) -> (x-y=w2249:dbl[])
                  }
                  frame True {
                    n452 = Add(x=w2251, y=w2252) -> (x+y=w2250:dbl[])
                  }
                }
                n453 = Multiply(x=w2195, y=6.283185307179586) -> (x*y=w2197:dbl)
                n454 = Sine(x=w2197) -> (sin(x)=w2201:dbl)
                n455 = Cosine(x=w2197) -> (cos(x)=w2202:dbl)
                n456 = Negate(x=w2201) -> (-x=w2198:dbl)
                n457 = Not(x=w2109) -> (.not. x?=w2107:bool)
                n458 = Build Array(w2202, w2198) -> (w2199:dbl[])
                n459 = Build Array(w2201, w2202) -> (w2200:dbl[])
                n460 = Build Array(w2199, w2200) -> (w2178:dbl[][])
                n461 = Bundle("sample mode"=w2170, "sample mode"=w2170) -> (w2171:cluster{"sample mode":i32, "sample mode":i32})  [unwired: 1 in]
                n462 = call-poly <vilib>:"A x B.vi"("B"=w2148, "A"=w2178) -> ("A x B"=w2147:T15)  [unwired: 1 out]
                n463 = In Range and Coerce(upper limit=0.0 ("element"), x=w2131, lower limit=10.0 ("element")) -> (coerced(x)=w2144:dbl[])  [unwired: 1 out]
                n464 = Divide(x=w2147, y=w2123) -> (x/y=w2146:T15)
                n465 = Array Size(array=w2144) -> (size(s)=w2143:i32)
                n466 = case shown="False" w2109 {
                  tunnel: w2173 -> [w2226 w2234]
                  tunnel: [w2225 w2233] -> w2172
                  tunnel: w2110 -> [w2224 w2232]
                  frame True {
                    n467 = Concatenate Strings(w2224, tag "/ao0," ("physical channels"), w2224, tag "/ao1," ("physical channels"), w2224, tag "/ao2" ("physical channels")) -> (w2221:string)
                    n468 = Type Cast(type=w2226, x=w2221) -> (*(type *) &x=w2225:tag)
                  }
                  frame False {
                    n469 = Concatenate Strings(w2232, tag "/ao0," ("physical channels"), w2232, tag "/ao1," ("physical channels"), w2232, tag "/ao2," ("physical channels"), w2232, tag "/ao3" ("physical channels")) -> (w2229:string)
                    n470 = Type Cast(type=w2234, x=w2229) -> (*(type *) &x=w2233:tag)
                  }
                }
                n471 = Index Array(array=w2146, index (row)=0 ("disabled index (col)")) -> (element=w2193:dbl[])  [unwired: 1 in]
                n472 = Index Array(array=w2146, index (row)=1 ("disabled index (col)")) -> (element=w2192:dbl[])  [unwired: 1 in]
                n473 = Multiply(x=w2143, y=15) -> (x*y=w2138:i32)
                n474 = Divide(x=w2138, y=360.0) -> (x/y=w2139:dbl)
                n475 = Add(x=w2192, y="y jog") -> (x+y=w2184:dbl[])
